vi "M02 Wind Turbine.vi"(11 "NXT/EV3":T1) -> (3 "EV3 out":T1)   [LabVIEW 2016]
uses:
  <vilib>/NXT/Subs/LVHSConnector.ctl
  <vilib>/NXT/LegoClasses/BrickReference/BrickReference.lvclass
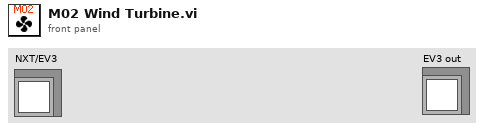
[diagram p1: front panel]
types:
  T1 = typedef "LVHSConnector.ctl" = refnum<class "BrickReference.lvclass">
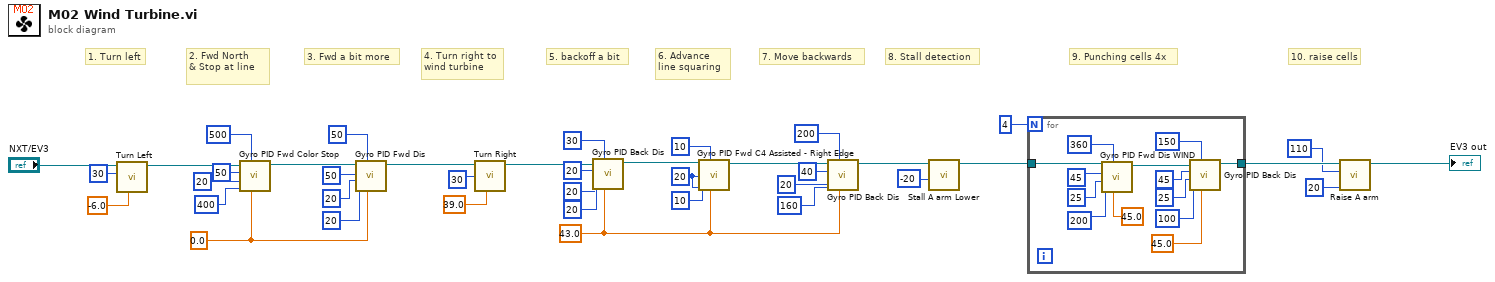
[diagram p0: block diagram]
diagram:
  w11 = sgl 0.0 ("Target angle")
  w9 = sgl 43.0 ("Target angle")
  w10 = 20 ("Max. speed")
  # "10. raise cells"
  # "9. Punching cells 4x"
  # "8. Stall detection"
  # "5. backoff a bit"
  # "7. Move backwards"
  # "6. Advance\nline squaring"
  # "4. Turn right to\nwind turbine"
  # "3. Fwd a bit more"
  # "2. Fwd North\n& Stop at line"
  # "1. Turn left"
  n1 = call "Turn Left.vi"("Turning angle"=sgl -6.0, "Motor B (right)"=i8 30, "EV3 in"="NXT/EV3") -> ("EV3 out"=w34:T1)  [unwired: 8 in]
  n2 = call "Gyro PID Fwd Color Stop.vi"("Target angle"=w11, "Threshold to Color"=500 ("Threshold to stop"), "Threshold to slow"=400, "Min. speed"=20, "Max. speed"=50, "EV3 in"=w34) -> ("EV3 out"=w21:T1)  [unwired: 5 in]
  n3 = call "Gyro PID Fwd Dis.vi"("Target angle"=w11, "Threshold to stop"=50, "Threshold to slow"=20, "Min. speed"=20, "Max. speed"=50, "EV3 in"=w21) -> ("EV3 out"=w20:T1)  [unwired: 5 in]
  n4 = call "Turn Right.vi"("Turning angle"=sgl 39.0, "Motor B (right)"=i8 30, "EV3 in"=w20) -> ("EV3 out"=w14:T1)  [unwired: 8 in]
  n5 = call "Gyro PID Back Dis.vi"("Target angle"=w9, "Threshold to stop"=30, "Threshold to slow"=20, "Min. speed"=20, "Max. speed"=20, "EV3 in"=w14) -> ("EV3 out"=w13:T1)  [unwired: 5 in]
  n6 = call "Gyro PID Fwd C4 Assisted - Right Edge.vi"("Target angle"=w9, "Threshold to Color"=10, "Threshold to slow"=w10, "Min. speed"=10, "Max. speed"=w10, "EV3 in"=w13) -> ("EV3 out"=w19:T1)  [unwired: 5 in]
  n7 = call "Gyro PID Back Dis.vi"("Target angle"=w9, "Threshold to stop"=200, "Threshold to slow"=160, "Min. speed"=20, "Max. speed"=40, "EV3 in"=w19) -> ("EV3 out"=w2:T1)  [unwired: 5 in]
  n8 = call "Stall A arm Lower.vi"("Power"=i8 -20, "NXT/EV3"=w2) -> ("NXT/EV3"=w7:T1)  [unwired: 9 in]
  n9 = for {
    N: 4 -> [_]
    tunnel: w7 -> [w43]
    tunnel: [w42] -> w5
    n10 = call "Gyro PID Fwd Dis WIND.vi"("Target angle"=sgl 45.0, "Threshold to stop"=360, "Threshold to slow"=200, "Higher speed"=25 ("Min. speed"), "Max. speed"=45, "EV3 in"=w43) -> ("EV3 out"=w41:T1)  [unwired: 5 in]
    n11 = call "Gyro PID Back Dis.vi"("Target angle"=sgl 45.0, "Threshold to stop"=150, "Threshold to slow"=100, "Min. speed"=25, "Max. speed"=45, "EV3 in"=w41) -> ("EV3 out"=w42:T1)  [unwired: 5 in]
  }
  n12 = call "Raise A arm.vi"("Power"=i8 20, "Rotation"=110, "EV3 in"=w5) -> ("EV3 out"=→"EV3 out":T1)  [unwired: 8 in]
